vi "周期启动 (子VI).vi"   [LabVIEW 2016, in "质控单元.lvlib"]
types:
  T1 = cluster{"是否启用仪器":bool, "CODMn":cluster{"启动测量模式":cluster{"测量模式":enum16{"水样测量", "标样核查", "加标回收", "平行样", "校零", "校标"}}, "确定按钮":bool}, "启动模块":cluster{"氨氮":bool, "总磷":bool, "总氮":bool, "CODMn":bool, "CODCr":bool}, "常规启动":bool, "直接启动":bool}
  T2 = cluster{"周期设置类型":enum16{"定点启动", "间隔启动"}, "定时功能启用":bool, "定时间隔":dbl, "间隔启动次数 ":dbl, "已经启动次数 ":dbl, "24H周期设置":bool[], "模块选择":cluster{"氨氮":bool, "总磷":bool, "总氮":bool, "CODMn":bool, "CODCr":bool}, "采配水启用":bool}
  T3 = typedef "LVDateTimeRec.ctl" = cluster{"秒数的小数部分":dbl, "秒":i32, "分":i32, "时":i32, "日":i32, "月":i32, "年":i32, "天数（周）":i32, "天数（年）":i32, "DST":i32}
  T4 = cluster{"氨氮":bool, "总磷":bool, "总氮":bool, "CODMn":bool, "CODCr":bool}
  T5 = enum32{"Bad", "Idle", "Run top level", "Running"}
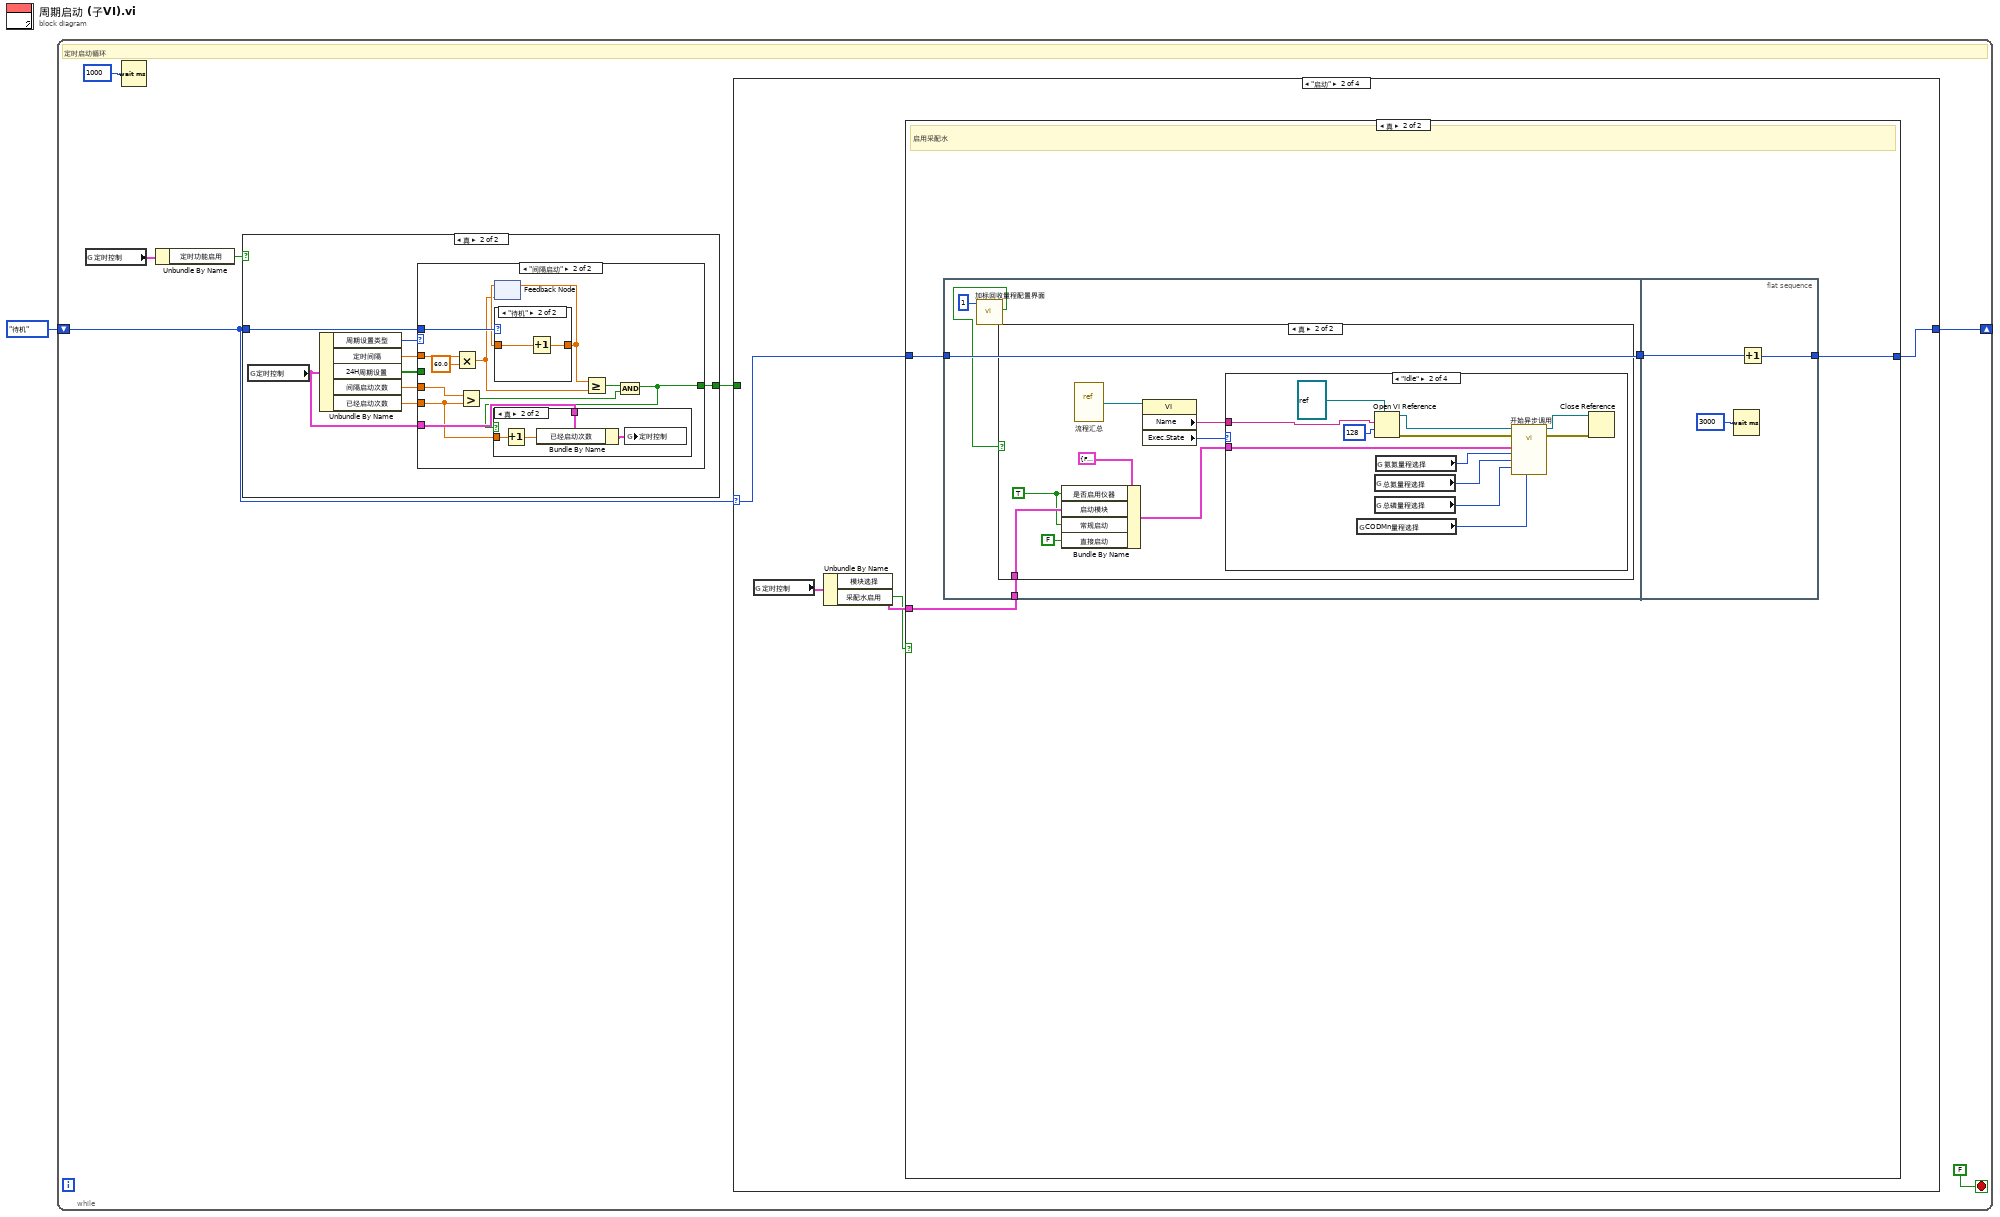
[diagram p0: block diagram]
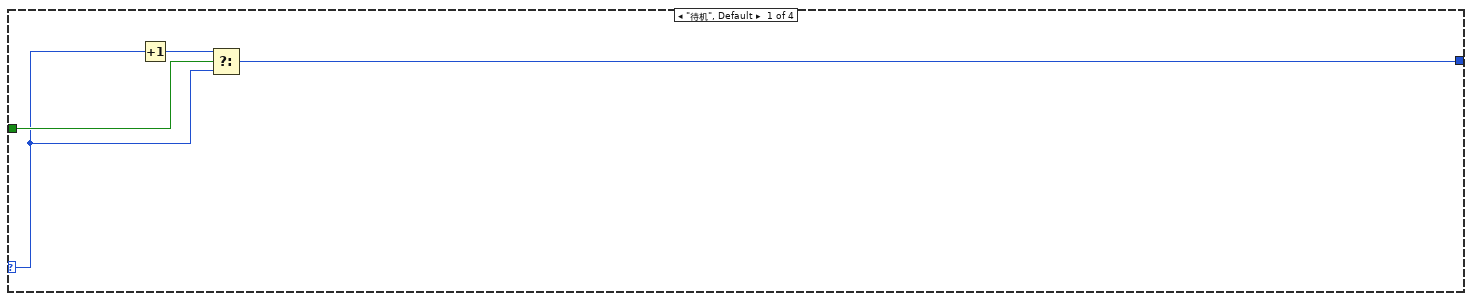
[diagram p2: hidden frame]
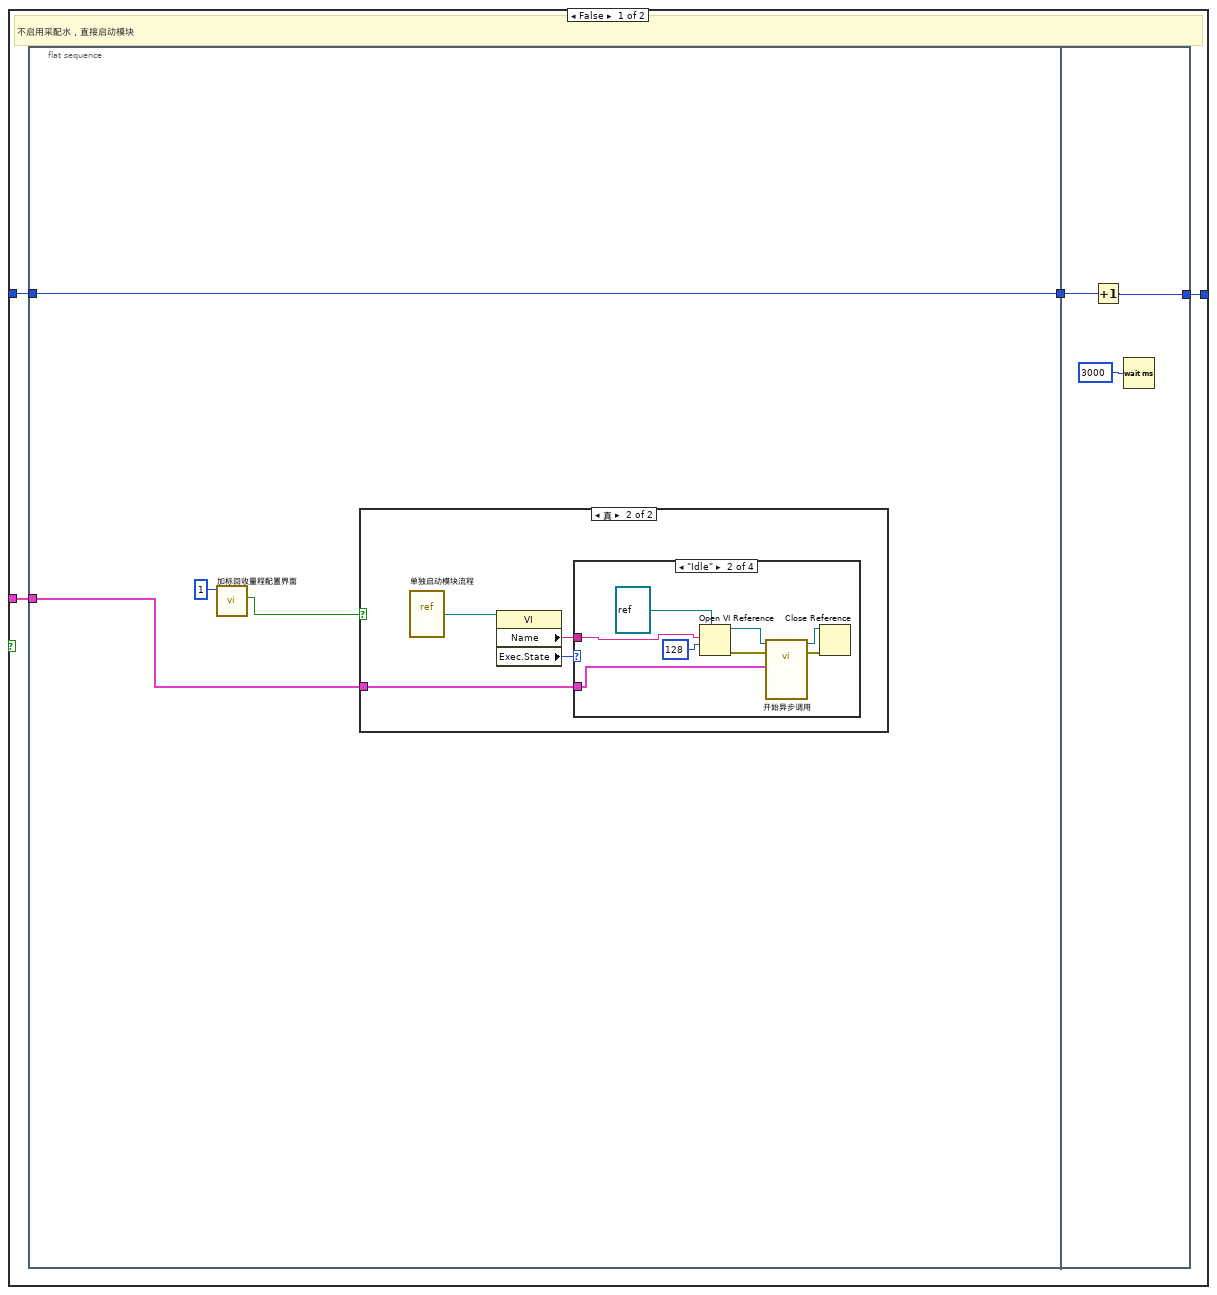
[diagram p3: hidden frame]
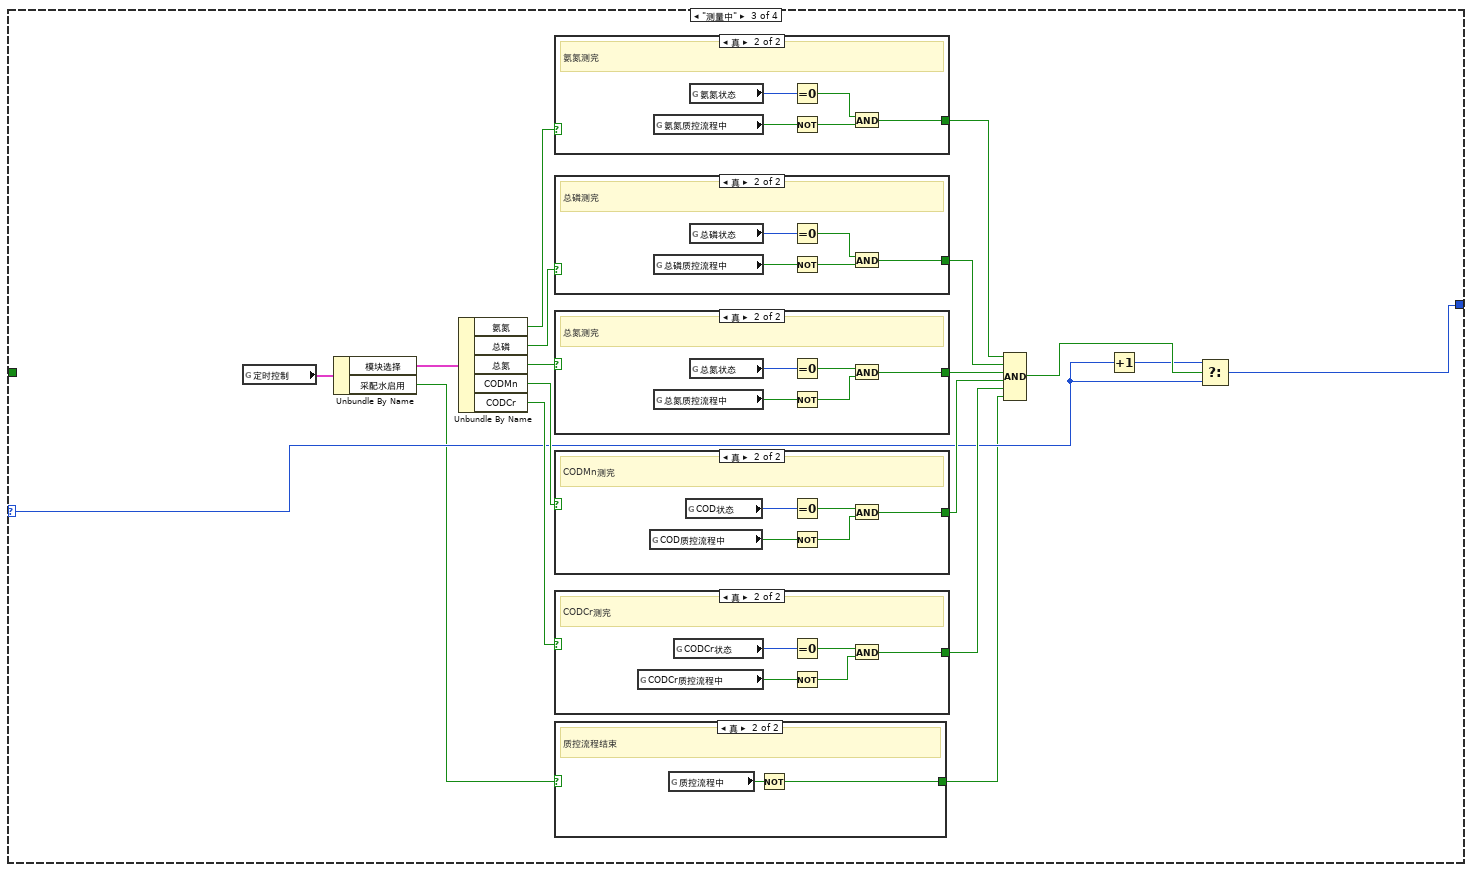
[diagram p12: hidden frame]
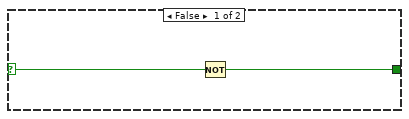
[diagram p13: hidden frame]
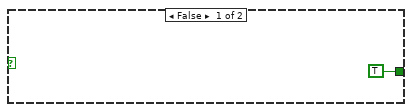
[diagram p14: hidden frame]
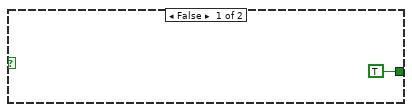
[diagram p15: hidden frame]
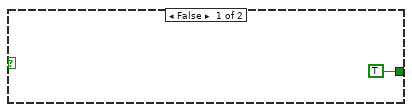
[diagram p16: hidden frame]
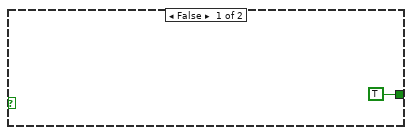
[diagram p17: hidden frame]
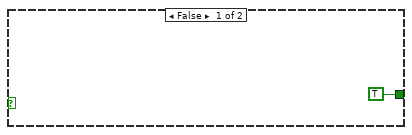
[diagram p18: hidden frame]
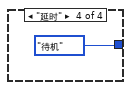
[diagram p19: hidden frame]
diagram:
  n1 = while {
    shift-right: [w6] -> _
    shift-left: enum16{"待机", "启动", "测量中", "延时"}."待机" -> [w5]
    stop <- FALSE stop-if-true
    # "定时启动循环"
    n2 = global read "断电保存全局.vi" "定时控制"() -> (w3:T2)
    n3 = Wait (ms)(milliseconds to wait=u32 1000 ("等待时间（毫秒）")) -> ()  [unwired: 1 out]
    n4 = Unbundle By Name(w3) -> ("定时功能启用"=w2:bool)
    n5 = case shown="真" w2 {
      tunnel: w5 -> [_ w129]
      tunnel: [_ w128] -> w4
      frame False {
      }
      frame True {
        n6 = global read "断电保存全局.vi" "定时控制"() -> (w125:T2)
        n7 = Unbundle By Name(w125) -> ("周期设置类型"=w130:enum16{"定点启动", "间隔启动"}, "定时间隔"=w131:dbl, "24H周期设置"=w132:bool[], "间隔启动次数"=w127:dbl, "已经启动次数"=w126:dbl)
        n8 = case shown="\"间隔启动\"" w130 {
          tunnel: w131 -> [_ w152]
          tunnel: w132 -> [w135 _]
          tunnel: w129 -> [w133 w155]
          tunnel: [w134 w144] -> w128
          tunnel: w127 -> [_ w148]
          tunnel: w126 -> [_ w145]
          tunnel: w125 -> [_ w146]
          frame "定点启动", Default {
            n9 = case shown="\"待机\", 默认" w133 {
              tunnel: w135 -> [w141 _]
              tunnel: [w136 _] -> w134
              frame "待机", Default {
                n10 = Get Date/Time In Seconds() -> (seconds since 1Jan1904=w143:timestamp)
                n11 = Seconds To Date/Time(time stamp (now)=w143) -> (date time rec=w142:T3)  [unwired: 1 in]
                n12 = Unbundle By Name(w142) -> ("时"=w140:i32, "分"=w139:i32)  [unwired: 1 out]
                n13 = Equal To 0?(x=w139) -> (x = 0?=w137:bool)
                n14 = Index Array(array=w141, index=w140) -> (element=w138:bool)
                n15 = Compound Arithmetic op=AND ("复合运算")(w138, w137) -> (w136:bool)
              }
              frame "启动" {
              }
            }
          }
          frame "间隔启动" {
            n16 = Multiply(x=w152, y=60.0) -> (x*y=w149:dbl)
            n17 = Greater?(x=w148, y=w145) -> (0:w147:bool)
            n18 = feedback #1(w149) -> (w154:dbl)
            n19 = case shown="\"待机\"" w155 {
              tunnel: w154 -> [_ w161]
              tunnel: [_ w160] -> w153
              frame Default {
              }
              frame "待机" {
                n20 = Increment(x=w161) -> (x+1=w160:dbl)
              }
            }
            n21 = feedback-in #1(w153) -> ()
            n22 = Greater Or Equal?(x=w153, y=w149) -> (x >= y?=w150:bool)
            n23 = And(x=w150, y=w147) -> (x .and. y?=w144:bool)
            n24 = case shown="真" w144 {
              tunnel: w146 -> [_ w159]
              tunnel: w145 -> [_ w158]
              frame False {
              }
              frame True {
                n25 = Increment(x=w158) -> (x+1=w157:dbl)
                n26 = Bundle By Name(cluster=w159, "已经启动次数"=w157) -> (w156:T2)
                n27 = global write "断电保存全局.vi" "定时控制"(w156) -> ()
              }
            }
          }
        }
      }
    }
    n28 = case shown="\"启动\"" w5 {
      selector: w5 -> [w9 w14 w75 _]
      tunnel: [w11 w17 w76 enum16{"待机", "启动", "测量中", "延时"}."待机"] -> w6
      tunnel: w4 -> [w12 _ _ _]
      frame "待机", Default {
        n29 = Increment(x=w9) -> (x+1=w10:enum16{"待机", "启动", "测量中", "延时"})
        n30 = Select(t=w10, s=w12, f=w9) -> (s? t:f=w11:enum16{"待机", "启动", "测量中", "延时"})
      }
      frame "启动" {
        n31 = global read "断电保存全局.vi" "定时控制"() -> (w15:T2)
        n32 = Unbundle By Name(w15) -> ("模块选择"=w16:T4, "采配水启用"=w13:bool)
        n33 = case shown="真" w13 {
          tunnel: [w20 w41] -> w17
          tunnel: w16 -> [w19 w44]
          tunnel: w14 -> [w18 w42]
          frame False {
            # "不启用采配水，直接启动模块"
            n34 = flat-sequence {
              tunnel: w19 -> [w24]
              tunnel: w18 -> [w25]
              tunnel: [w25] -> w21
              tunnel: [w40] -> w20
              tunnel: w21 -> [w39]
              frame #0 {
                n35 = call "加标回收量程配置界面.vi"("倒计时"=u16 1) -> ("布尔"=w22:bool)  [unwired: 9 in, 1 out]
                n36 = case shown="真" w22 {
                  tunnel: w24 -> [_ w26]
                  frame False {
                  }
                  frame True {
                    n37 = vi-ref "单独启动模块流程.vi"() -> (w27:refnum<vi>)
                    n38 = property class="VI"(reference=w27) -> ("Name"=w29:string, "Exec.State"=w28:T5)  [unwired: 1 in, 2 out]
                    n39 = case shown="\"Idle\"" w28 {
                      tunnel: w29 -> [_ w33 _ _]
                      tunnel: w26 -> [_ w30 _ _]
                      frame "Bad", Default {
                      }
                      frame "Idle" {
                        n40 = Open VI Reference(type specifier VI Refnum (for type only)=refnum<vi> refnum ("类型说明符VI引用句柄（仅用于类型）"), vi path=w33, options=128 ("选项")) -> (vi reference=w37:refnum<vi>, error out=w32:errorcluster)  [unwired: 3 in]
                        n41 = call-by-ref "开始异步调用"(reference=w37, error in=w32, "模块选择"=w30) -> (reference out=w36:refnum<vi>, error out=w31:errorcluster)  [unwired: 11 in]
                        n42 = Close Reference(reference=w36, error in (no error)=w31) -> ()  [unwired: 1 out]
                      }
                      frame "Run top level" {
                      }
                      frame "Running" {
                      }
                    }
                  }
                }
              }
              frame #1 {
                n43 = Increment(x=w39) -> (x+1=w40:enum16{"待机", "启动", "测量中", "延时"})
                n44 = Wait (ms)(milliseconds to wait=u32 3000 ("等待时间（毫秒）")) -> ()  [unwired: 1 out]
              }
            }
          }
          frame True {
            # "启用采配水"
            n45 = flat-sequence {
              tunnel: w44 -> [w48]
              tunnel: [w47] -> w43
              tunnel: w42 -> [w47]
              tunnel: w43 -> [w71]
              tunnel: [w70] -> w41
              frame #0 {
                n46 = call "加标回收量程配置界面.vi"("倒计时"=u16 1) -> ("布尔"=w45:bool)  [unwired: 9 in, 1 out]
                n47 = case shown="真" w45 {
                  tunnel: w48 -> [_ w52]
                  frame False {
                  }
                  frame True {
                    w51 = TRUE ("是否启用仪器")
                    n48 = Bundle By Name(cluster=T1 {"是否启用仪器"=FALSE, "CODMn"={"启动测量模式"={"测量模式"=enum."水样测量"}, "确定按钮"=FALSE}, "启动模块"={"氨氮"=FALSE, "总磷"=FALSE, "总氮"=FALSE, "CODMn"=FALSE, "CODCr"=FALSE}, "常规启动"=FALSE, "直接启动"=FALSE} ("参数"), "是否启用仪器"=w51, "启动模块"=w52, "常规启动"=w51, "直接启动"=FALSE) -> (w49:T1)
                    n49 = vi-ref "流程汇总.vi"() -> (w55:refnum<vi>)
                    n50 = property class="VI"(reference=w55) -> ("Name"=w56:string, "Exec.State"=w54:T5)  [unwired: 1 in, 2 out]
                    n51 = case shown="\"Idle\"" w54 {
                      tunnel: w56 -> [_ w67 _ _]
                      tunnel: w49 -> [_ w57 _ _]
                      frame "Bad", Default {
                      }
                      frame "Idle" {
                        n52 = global read "断电保存全局.vi" "CODMn量程选择"() -> (w61:enum32{"H", "L", "AUTO"})
                        n53 = Open VI Reference(type specifier VI Refnum (for type only)=refnum<vi> refnum ("类型说明符VI引用句柄（仅用于类型）"), vi path=w67, options=128 ("选项")) -> (vi reference=w68:refnum<vi>, error out=w64:errorcluster)  [unwired: 3 in]
                        n54 = global read "断电保存全局.vi" "总氮量程选择"() -> (w59:enum32{"H", "L", "AUTO"})
                        n55 = global read "断电保存全局.vi" "总磷量程选择"() -> (w60:enum32{"H", "L", "AUTO"})
                        n56 = global read "断电保存全局.vi" "氨氮量程选择"() -> (w58:enum32{"H", "L", "AUTO"})
                        n57 = call-by-ref "开始异步调用"(reference=w68, error in=w64, "CODMn量程切换"=w61, "总磷量程切换"=w60, "总氮量程切换"=w59, "氨氮量程切换"=w58, "参数"=w57) -> (reference out=w66:refnum<vi>, error out=w65:errorcluster)  [unwired: 7 in]
                        n58 = Close Reference(reference=w66, error in (no error)=w65) -> ()  [unwired: 1 out]
                      }
                      frame "Run top level" {
                      }
                      frame "Running" {
                      }
                    }
                  }
                }
              }
              frame #1 {
                n59 = Wait (ms)(milliseconds to wait=u32 3000 ("等待时间（毫秒）")) -> ()  [unwired: 1 out]
                n60 = Increment(x=w71) -> (x+1=w70:enum16{"待机", "启动", "测量中", "延时"})
              }
            }
          }
        }
      }
      frame "测量中" {
        n61 = global read "断电保存全局.vi" "定时控制"() -> (w89:T2)
        n62 = Unbundle By Name(w89) -> ("模块选择"=w88:T4, "采配水启用"=w74:bool)
        n63 = Unbundle By Name(w88) -> ("氨氮"=w81:bool, "总磷"=w80:bool, "总氮"=w79:bool, "CODMn"=w78:bool, "CODCr"=w77:bool)
        n64 = case shown="真" w81 {
          tunnel: [TRUE w121] -> w82
          frame False {
          }
          frame True {
            # "氨氮测完"
            n65 = global read "质控测完标志全局 1.vi" "氨氮质控流程中"() -> (w123:bool)
            n66 = global read "加标回收状态全局变量.vi" "氨氮状态"() -> (w120:u16)
            n67 = Equal To 0?(x=w120) -> (x = 0?=w119:bool)
            n68 = Not(x=w123) -> (.not. x?=w122:bool)
            n69 = And(x=w119, y=w122) -> (x .and. y?=w121:bool)
          }
        }
        n70 = case shown="真" w80 {
          tunnel: [TRUE w115] -> w83
          frame False {
          }
          frame True {
            # "总磷测完"
            n71 = global read "质控测完标志全局 1.vi" "总磷质控流程中"() -> (w117:bool)
            n72 = global read "加标回收状态全局变量.vi" "总磷状态"() -> (w114:u16)
            n73 = Equal To 0?(x=w114) -> (x = 0?=w113:bool)
            n74 = Not(x=w117) -> (.not. x?=w116:bool)
            n75 = And(x=w113, y=w116) -> (x .and. y?=w115:bool)
          }
        }
        n76 = case shown="真" w79 {
          tunnel: [TRUE w109] -> w84
          frame False {
          }
          frame True {
            # "总氮测完"
            n77 = global read "质控测完标志全局 1.vi" "总氮质控流程中"() -> (w111:bool)
            n78 = global read "加标回收状态全局变量.vi" "总氮状态"() -> (w108:u16)
            n79 = Equal To 0?(x=w108) -> (x = 0?=w107:bool)
            n80 = Not(x=w111) -> (.not. x?=w110:bool)
            n81 = And(x=w107, y=w110) -> (x .and. y?=w109:bool)
          }
        }
        n82 = case shown="真" w78 {
          tunnel: [TRUE w103] -> w85
          frame False {
          }
          frame True {
            # "CODMn测完"
            n83 = global read "质控测完标志全局 1.vi" "COD质控流程中"() -> (w105:bool)
            n84 = global read "加标回收状态全局变量.vi" "COD状态"() -> (w102:u16)
            n85 = Equal To 0?(x=w102) -> (x = 0?=w101:bool)
            n86 = Not(x=w105) -> (.not. x?=w104:bool)
            n87 = And(x=w101, y=w104) -> (x .and. y?=w103:bool)
          }
        }
        n88 = case shown="真" w77 {
          tunnel: [TRUE w97] -> w86
          frame False {
          }
          frame True {
            # "CODCr测完"
            n89 = global read "质控测完标志全局 1.vi" "CODCr质控流程中"() -> (w99:bool)
            n90 = global read "加标回收状态全局变量.vi" "CODCr状态"() -> (w96:u16)
            n91 = Equal To 0?(x=w96) -> (x = 0?=w95:bool)
            n92 = Not(x=w99) -> (.not. x?=w98:bool)
            n93 = And(x=w95, y=w98) -> (x .and. y?=w97:bool)
          }
        }
        n94 = case shown="真" w74 {
          selector: w74 -> [w91 _]
          tunnel: [w90 w92] -> w73
          frame False {
            n95 = Not(x=w91) -> (.not. x?=w90:bool)
          }
          frame True {
            # "质控流程结束"
            n96 = global read "质控测完标志全局 1.vi" "质控流程中"() -> (w93:bool)
            n97 = Not(x=w93) -> (.not. x?=w92:bool)
          }
        }
        n98 = Compound Arithmetic op=AND ("复合运算")(w82, w83, w84, w85, w86, w73) -> (w87:bool)
        n99 = Increment(x=w75) -> (x+1=w72:enum16{"待机", "启动", "测量中", "延时"})
        n100 = Select(t=w72, s=w87, f=w75) -> (s? t:f=w76:enum16{"待机", "启动", "测量中", "延时"})
      }
      frame "延时" {
      }
    }
  }
